vi "Update Root Message.vi"(8 "error in (no error)":errorcluster, 10 "Message":string, 11 "Root Interface in":refnum<class "Root Interface.lvclass">) -> (0 "error out":errorcluster, 3 "Root Interface out":refnum<class "Root Interface.lvclass">)   [LabVIEW 2025, in "Root Interface.lvlib" / "Root Interface.lvclass"]
uses:
  Root Interface.lvclass
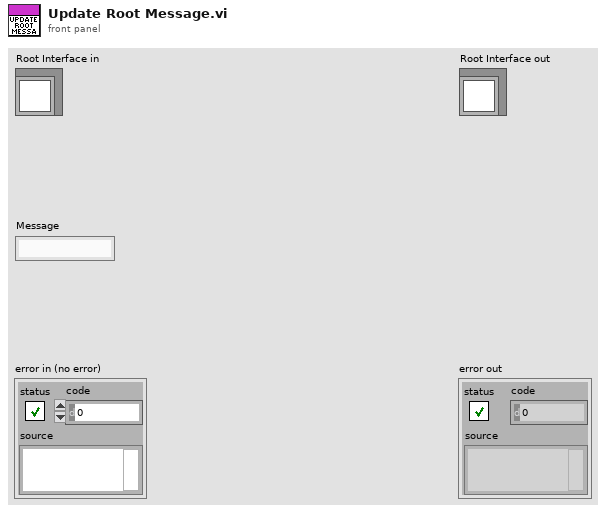
[diagram p1: front panel]
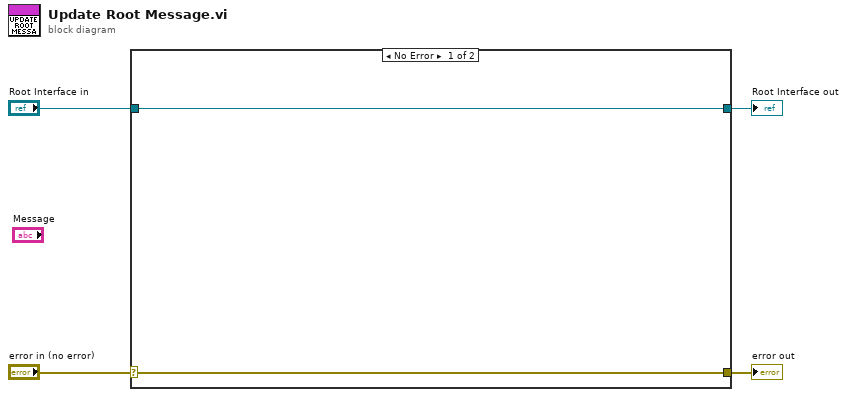
[diagram p0: block diagram]
diagram:
  n1 = case shown="No Error" "error in (no error)" {
    selector: "error in (no error)" -> [w5 w8]
    tunnel: [w5 w8] -> w3
    tunnel: [w6 w7] -> w1
    tunnel: "Root Interface in" -> [w6 w7]
    frame No Error {
    }
    frame Error {
    }
  }
  "error out" <- w3
  "Root Interface out" <- w1
